vi "n64_generate_grid.vi"(6 "Reset":bool=TRUE, 8 "Tare":bool=TRUE, 9 "Row Length":i32=64, 10 "No. Nodes":i32=64, 11 "Sensor Readings (PACKET)":i16[](array[numeric])) -> (0 "Node XYZ List":dbl[][](array[numeric]), 1 "Y (GRID)":dbl[][](array[numeric]), 2 "X (GRID)":dbl[][](array[numeric]), 3 "Z (GRID)":dbl[][](array[numeric]), 4 "Mag_GRID":dbl[][](array[numeric]))   [LabVIEW 2016]
panel:
  in  "Tab Control":enum32{"16 Node", "64 Node"}(tab)
  in  "Lookup Index n16":i32[](array[numeric])=[0, 2, 1, 3, 4, 6, 5, 7, 8, 10, 9, 11, 12, 14, 13, 15]
  in  "Inv Gain n16":i32[][](array[numeric])=[[1, 1, 1], [1, 1, -1], [1, 1, 1], [1, 1, 1], [1, 1, 1], [1, 1, -1], [1, 1, -1], [1, 1, -1], [1, 1, -1], [1, 1, -1], [1, 1, -1], [1, 1, 1], [1, 1, -1], [1, 1, 1], [1, 1, 1], [1, 1, -1]]
  in  "Lookup Index n64":i32[](array[numeric])=[0, 1, 2, 3, 4, 5, 6, 7, 15, 14, 13, 12, 11, 10, 9, 8, 16, 17, 18, 19, 20, 21, 22, 23, 31, 30, 29, 28, 27, 26, 25, 24, 32, 33, 34, 35, 36, 37, 38, 39, 47, 46, 45, 44, 43, 42, 41, 40, 55, 54, 53, 52, 51, 50, 49, 48, 63, 62, 61, 60, 59, 58, 57, 56]
  in  "Inv Gain n64":i32[][](array[numeric])=[[1, 1, 1], [1, 1, 1], [1, 1, 1], [1, 1, 1], [1, 1, 1], [1, 1, 1], [1, 1, 1], [1, 1, 1], [1, 1, 1], [1, 1, 1], [1, 1, 1], [1, 1, 1], [1, 1, 1], [1, 1, 1], [1, 1, 1], [1, 1, 1], [1, 1, 1], [1, 1, 1], [1, 1, 1], [1, 1, 1], [1, 1, 1], [1, 1, 1], [1, 1, 1], [1, 1, 1], [1, 1, 1], [1, 1, 1], [1, 1, 1], [1, 1, 1], [1, 1, 1], [1, 1, -1], [1, 1, 1], [1, 1, 1], [1, 1, 1], [1, 1, 1], [1, 1, 1], [1, 1, 1], [1, 1, 1], [1, 1, 1], [1, 1, 1], [1, 1, 1], [1, 1, 1], [1, 1, 1], [1, 1, 1], [1, 1, 1], [1, 1, 1], [1, 1, 1], [1, 1, 1], [1, 1, 1], [1, 1, 1], [1, 1, 1], [1, 1, 1], [1, 1, 1], [1, 1, 1], [1, 1, 1], [1, 1, 1], [1, 1, 1], [1, 1, 1], [1, 1, 1], [1, 1, 1], [1, 1, -1], [1, 1, -1], [1, 1, 1], [1, 1, 1], [1, 1, 1]]
  in  "Tare":dbl[][](array[numeric])=[[0.00018775, -0.000174232, 3312.98], [0.000139686, -0.00039953199999999997, 2906.42], [-0.000288384, -0.001229387, 2606.34], [-3.6799e-05, -0.0012016, 3702.6], [0.000266605, -0.001108476, 3847.7999999999997], [0.00038301, -0.000208027, 3472.7], [-0.000177236, -0.000316171, 3651.7799999999997], [-0.00024557699999999997, 0.000544475, 4767.4], [-5.6325e-05, -0.00041305, 4172.08], [8.4112e-05, 0.000956774, 2562.7799999999997], [-0.000261348, 0.001097962, 3675.98], [-0.00014944899999999998, -0.00066839, 4856.94], [-0.000204272, 0.000920726, 4740.78], [-0.000242573, -7.7353e-05, 4009.94], [0.000246328, -0.000138184, 4358.42], [7.51e-06, 0.000451351, 5829.78]]
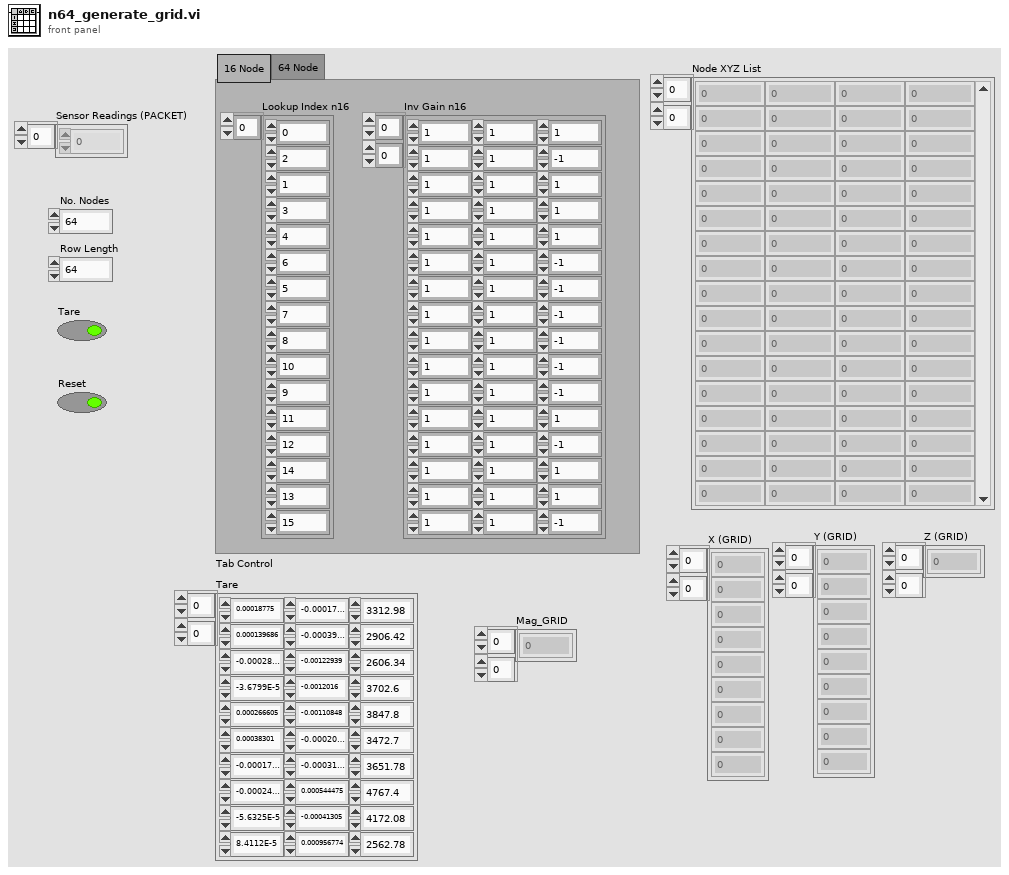
[diagram p1: front panel]
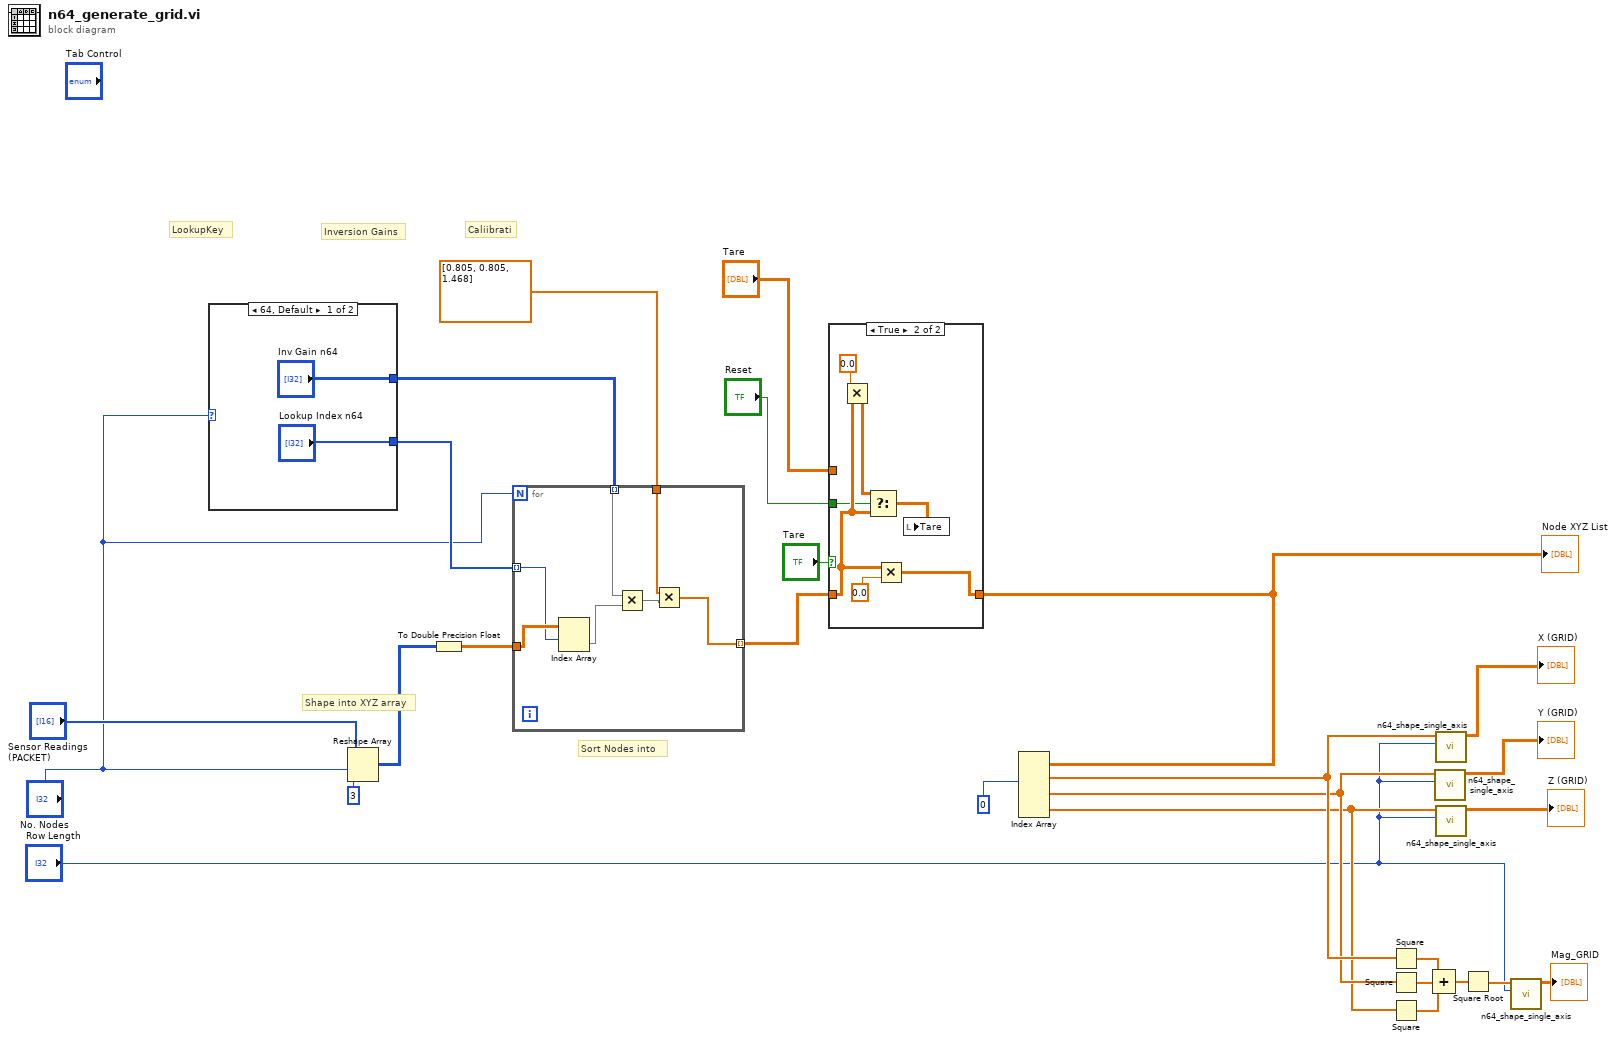
[diagram p0: block diagram]
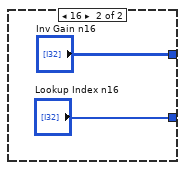
[diagram p2: hidden frame]
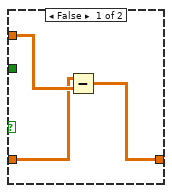
[diagram p3: hidden frame]
diagram:
  # "Caliibrati"
  # "Inversion Gains"
  # "LookupKey"
  # "Sort Nodes into"
  # "Shape into XYZ array"
  n1 = case shown="64, Default" "No. Nodes" {
    tunnel: ["Lookup Index n64" "Lookup Index n16"] -> w24
    tunnel: ["Inv Gain n64" "Inv Gain n16"] -> w22
    frame 64, Default {
    }
    frame 16 {
    }
  }
  n2 = Reshape Array("Sensor Readings (PACKET)", "No. Nodes", 3 ("milliseconds to wait")) -> (w21:i16[][])
  n3 = To Double Precision Float(number=w21) -> (double precision float=w20:dbl[][])
  n4 = for {
    N: "No. Nodes" -> [_]
    tunnel: w20 -> [w38]
    tunnel: w24 -> [w32] mode=indexing
    tunnel: [w33] -> w19 mode=indexing
    tunnel: dbl[] [0.805, 0.805, 1.468] -> [w35]
    tunnel: w22 -> [w37] mode=indexing
    n5 = Index Array(array=w38, index (row)=w32) -> (element=w34:dbl[])  [unwired: 1 in]
    n6 = Multiply(x=w37, y=w34) -> (x*y=w36:dbl[])
    n7 = Multiply(x=w35, y=w36) -> (x*y=w33:dbl[])
  }
  n8 = case shown="True" "Tare" {
    tunnel: w19 -> [w39 w45]
    tunnel: [w41 w47] -> w18
    tunnel: "Tare" -> [w40 _]
    tunnel: "Reset" -> [_ w42]
    frame False {
      n9 = Subtract(x=w39, y=w40) -> (x-y=w41:dbl[][])
    }
    frame True {
      n10 = Multiply(x=0.0 ("milliseconds to wait"), y=w45) -> (x*y=w44:dbl[][])
      n11 = Select(t=w44, s=w42, f=w45) -> (s? t:f=w46:dbl[][])
      n12 = Multiply(x=w45, y=0.0 ("milliseconds to wait")) -> (x*y=w47:dbl[][])
      n13 = local write "Tare"(w46) -> ()
    }
  }
  "Node XYZ List" <- w18
  n14 = Index Array(array=w18, index (col) #1=0 ("disabled index (col)")) -> (element #1=w14:dbl[], element #2=w13:dbl[], element #3=w12:dbl[])  [unwired: 5 in]
  n15 = Square(x=w14) -> (x^2=w11:dbl[])
  n16 = Square(x=w13) -> (x^2=w9:dbl[])
  n17 = Square(x=w12) -> (x^2=w10:dbl[])
  n18 = Compound Arithmetic op=ADD(w11, w9, w10) -> (w8:dbl[])
  n19 = call "n64_shape_single_axis.vi"("Row Length"="Row Length", "Readings (FLAT)"=w13) -> ("Readings (GRID)"=→"Y (GRID)":dbl[][])  [unwired: 9 in]
  n20 = call "n64_shape_single_axis.vi"("Row Length"="Row Length", "Readings (FLAT)"=w14) -> ("Readings (GRID)"=→"X (GRID)":dbl[][])  [unwired: 9 in]
  n21 = call "n64_shape_single_axis.vi"("Row Length"="Row Length", "Readings (FLAT)"=w12) -> ("Readings (GRID)"=→"Z (GRID)":dbl[][])  [unwired: 9 in]
  n22 = Square Root(x=w8) -> (sqrt(x)=w7:dbl[])
  n23 = call "n64_shape_single_axis.vi"("Row Length"="Row Length", "Readings (FLAT)"=w7) -> ("Readings (GRID)"=→"Mag_GRID":dbl[][])  [unwired: 9 in]
